vi "Get Ball Position.vi"(11 "Particle Measurements (Pixels)":dbl[][](array[numeric]) format="%.2f") -> (2 "Ball 2":dbl[](array[numeric]), 3 "Ball 1":dbl[](array[numeric]))   [LabVIEW 2014]
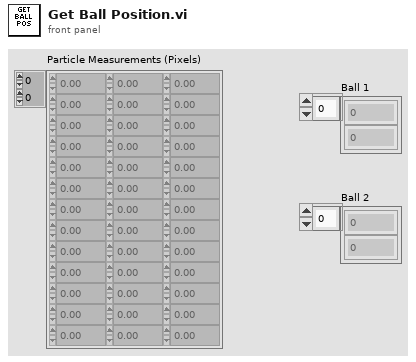
[diagram p1: front panel]
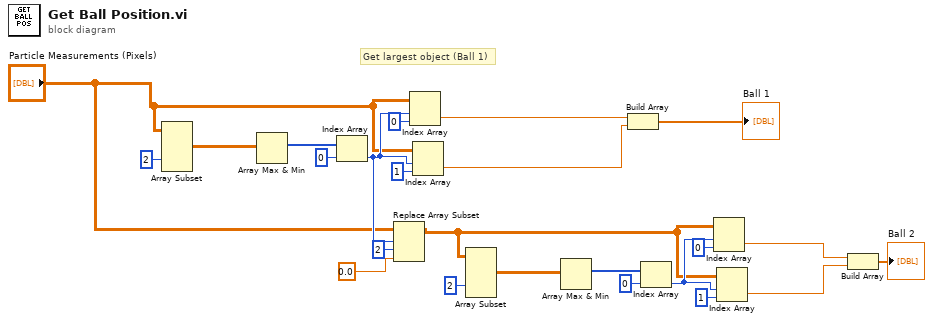
[diagram p0: block diagram]
diagram:
  # "Get largest object (Ball 1)"
  n1 = Array Subset(array="Particle Measurements (Pixels)", index (col)=2 ("index")) -> (w23:dbl[][])  [unwired: 3 in]
  n2 = Array Max & Min(array=w23) -> (max index (indices)=w19:i32[])  [unwired: 3 out]
  n3 = Index Array(array=w19, index=0) -> (element=w18:i32)
  n4 = Replace Array Subset(array="Particle Measurements (Pixels)", new element=0.0 ("new element/subarray"), index (row)=w18, index (col)=2 ("disabled index (col)")) -> (w7:dbl[][])
  n5 = Index Array(array="Particle Measurements (Pixels)", index (row)=w18, index (col)=0 ("disabled index (col)")) -> (element=w6:dbl)
  n6 = Index Array(array="Particle Measurements (Pixels)", index (row)=w18, index (col)=1 ("disabled index (col)")) -> (element=w5:dbl)
  n7 = Array Subset(array=w7, index (col)=2 ("index")) -> (w9:dbl[][])  [unwired: 3 in]
  n8 = Array Max & Min(array=w9) -> (max index (indices)=w13:i32[])  [unwired: 3 out]
  n9 = Build Array(w6, w5) -> (→"Ball 1":dbl[])
  n10 = Index Array(array=w13, index=0) -> (element=w14:i32)
  n11 = Index Array(array=w7, index (row)=w14, index (col)=0 ("disabled index (col)")) -> (element=w3:dbl)
  n12 = Index Array(array=w7, index (row)=w14, index (col)=1 ("disabled index (col)")) -> (element=w2:dbl)
  n13 = Build Array(w3, w2) -> (→"Ball 2":dbl[])
